vi "Lab4_3.vi"() -> ()   [LabVIEW 2011]
panel:
  out "Массив 2":dbl[](array[numeric])
  out "Массив 1":dbl[](array[numeric])
  out "Nmin":dbl
  out "Nmax":dbl
  in  "Кол-во\nитерация":i32
  in  "Число n":dbl
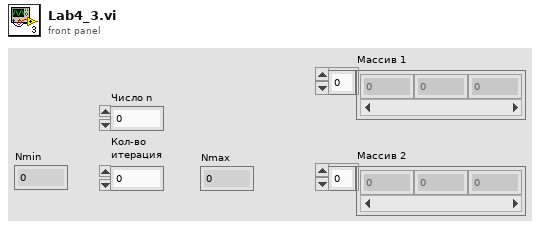
[diagram p1: front panel]
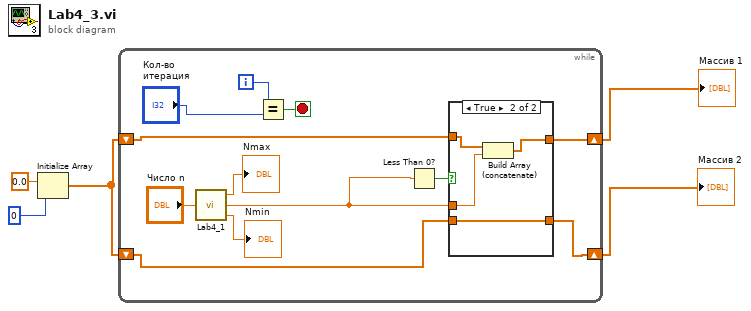
[diagram p0: block diagram]
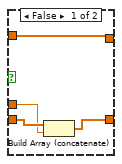
[diagram p2: hidden frame]
diagram:
  n1 = Initialize Array(0.0 ("element"), 0 ("dimension size")) -> (w3:dbl[])
  n2 = while {
    shift-right: [w10] -> w1
    shift-left: w3 -> [w13]
    shift-right: [w12] -> w2
    shift-left: w3 -> [w11]
    i -> [w8]
    stop <- w7 stop-if-true
    n3 = call "Lab4_1.vi"("n"="Число n") -> ("Nmin"=→"Nmin":dbl, "Результат"=w9:dbl, "Nmax"=→"Nmax":dbl)  [unwired: 2 in]
    n4 = Equal?(x=w8, y="Кол-во\nитерация") -> (x = y?=w7:bool)
    n5 = Less Than 0?(x=w9) -> (x < 0?=w14:bool)
    n6 = case shown="True" w14 {
      tunnel: w13 -> [w18 w25]
      tunnel: [w20 w24] -> w12
      tunnel: w11 -> [w21 w24]
      tunnel: [w18 w23] -> w10
      tunnel: w9 -> [w19 w22]
      frame False {
        n7 = Build Array (concatenate)(w21, w19) -> (w20:dbl[])
      }
      frame True {
        n8 = Build Array (concatenate)(w25, w22) -> (w23:dbl[])
      }
    }
  }
  "Массив 1" <- w1
  "Массив 2" <- w2
